vi "SAM-Init.vi"(0 "SAM In":T1, 11 "error in (no error)":errorcluster) -> (4 "SAM Out":T1, 15 "error out":errorcluster)   [LabVIEW 2020]
uses:
  SAM Params.ctl
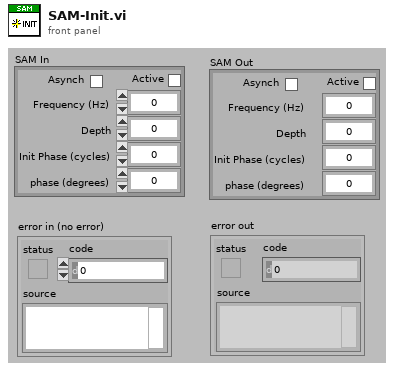
[diagram p1: front panel]
types:
  T1 = typedef "SAM Params.ctl" = cluster{"Active":bool, "Frequency (Hz)":dbl, "Depth":dbl, "Init Phase (cycles)":dbl, "phase (degrees)":dbl, "Asynch":bool}
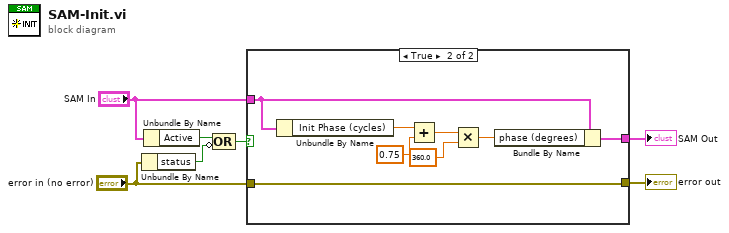
[diagram p0: block diagram]
diagram:
  n1 = Unbundle By Name("error in (no error)") -> ("status"=w4:bool)
  n2 = Unbundle By Name("SAM In") -> ("Active"=w5:bool)
  n3 = Compound Arithmetic op=OR(w5, invert w4) -> (w3:bool)
  n4 = case shown="True" w3 {
    tunnel: [w9 w10] -> w7
    tunnel: "error in (no error)" -> [w9 w10]
    tunnel: "SAM In" -> [w8 w13]
    tunnel: [w8 w11] -> w1
    frame False {
    }
    frame True {
      n5 = Unbundle By Name(w13) -> ("Init Phase (cycles)"=w15:dbl)
      n6 = Add(x=w15, y=0.75) -> (x+y=w17:dbl)
      n7 = Multiply(x=w17, y=360.0) -> (x*y=w12:dbl)
      n8 = Bundle By Name(cluster=w13, "phase (degrees)"=w12) -> (w11:T1)
    }
  }
  "error out" <- w7
  "SAM Out" <- w1
